vi "Mirror_Mode_DUAL_AE.vi"(2 "Action":T2, 7 "Mirror Modes In":T1) -> (8 "Mirror Modes Out":T1)   [LabVIEW 2014]
uses:
  Controls/Standard Action.ctl
  Controls/MirrorModes_DUAL.ctl
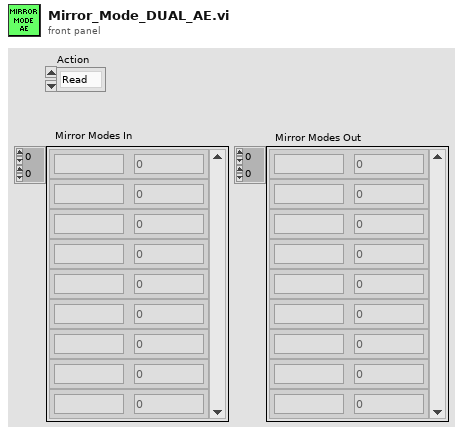
[diagram p1: front panel]
types:
  T1 = typedef "MirrorModes_DUAL.ctl" = cluster{"Mode":string, "Amplitude":dbl}[][]
  T2 = typedef "Standard Action.ctl" = enum16{"Read", "Write"}
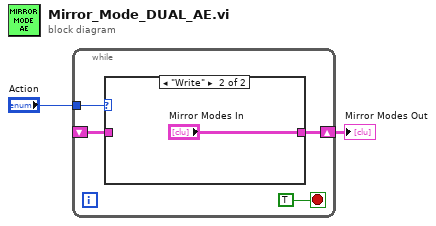
[diagram p0: block diagram]
diagram:
  n1 = while {
    tunnel: "Action" -> [w6]
    shift-right: [w5] -> w1
    shift-left: _ -> [w3]
    stop <- TRUE stop-if-true
    n2 = case shown="\"Write\"" w6 {
      tunnel: [w7 "Mirror Modes In"] -> w5
      tunnel: w3 -> [w7 _]
      frame "Read", Default {
      }
      frame "Write" {
      }
    }
  }
  "Mirror Modes Out" <- w1
